vi "Ballard XML Generator.Close Tx Channel.vi"(11 "string in":string) -> (3 "string out":string)   [LabVIEW 2017]
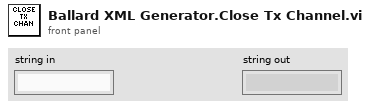
[diagram p1: front panel]
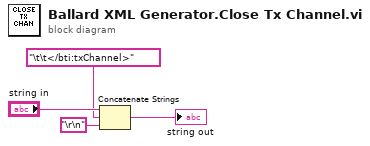
[diagram p0: block diagram]
diagram:
  n1 = Concatenate Strings("string in", "\t\t</bti:txChannel>", "\r\n") -> (→"string out":string)
